vi "Set 2D Next Vector_entwurf.vi"(0 "Coordinate System":u16(ring) items=["Cartesian", "Polar"], 1 "Magnetic Field Units":u16(ring) items=["kG", "Tesla"], 3 "User defined Ramp Rate (T/min)":dbl format="%.3f", 4 "Magnitude Limit (kG)":dbl format="%.3f", 5 "Y-Axis Communications Config":T1={"GPIB address"=22, "GPIB bus"=0, "connection ID"=refnum, "IP"="192.168.2.200", "Active Comm Interface"=0, "Serial Port"="", "Programmer Type"=0} {"Programmer Type" items=["Model 430", "Model 420"]; "Active Comm Interface" items=["TCP/IP (Model 430 Only)", "RS232", "IEEE488"]}, 6 "Input Vector":string[](array[string]), 7 "Z-Axis Communications Config":T1={"GPIB address"=22, "GPIB bus"=0, "connection ID"=refnum, "IP"="192.168.2.200", "Active Comm Interface"=0, "Serial Port"="", "Programmer Type"=0} {"Programmer Type" items=["Model 430", "Model 420"]; "Active Comm Interface" items=["TCP/IP (Model 430 Only)", "RS232", "IEEE488"]}, 10 "User defined Ramp Rate (T/min)":bool, 13 "Max Ramp Rate - Y Axis (A/s)":dbl format="%.3f", 14 "error in":T2, 15 "Max Ramp Rate - Z Axis (A/s)":dbl format="%.3f") -> (11 "Y-Axis Ramp Rate (T/min)":dbl format="%.3f", 12 "Within Limits?":bool, 16 "Ramp Rate along Vector (T/min)":dbl, 17 "Z-Axis Ramp Rate (T/min)":dbl format="%.3f", 18 "All Instruments Responded?":bool, 19 "error out":T2)   [LabVIEW 2016]
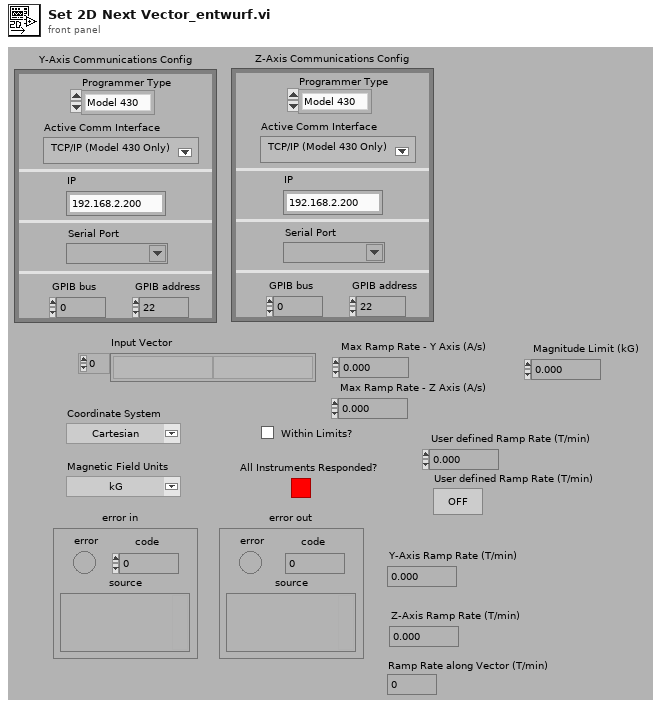
[diagram p1: front panel]
types:
  T1 = cluster{"GPIB address":i16, "GPIB bus":i16, "connection ID":refnum<k5>, "IP":string, "Active Comm Interface":u16, "Serial Port":refnum<visa-resource-name>, "Programmer Type":u16}
  T2 = cluster{"error":bool, "code":i32, "source":string}
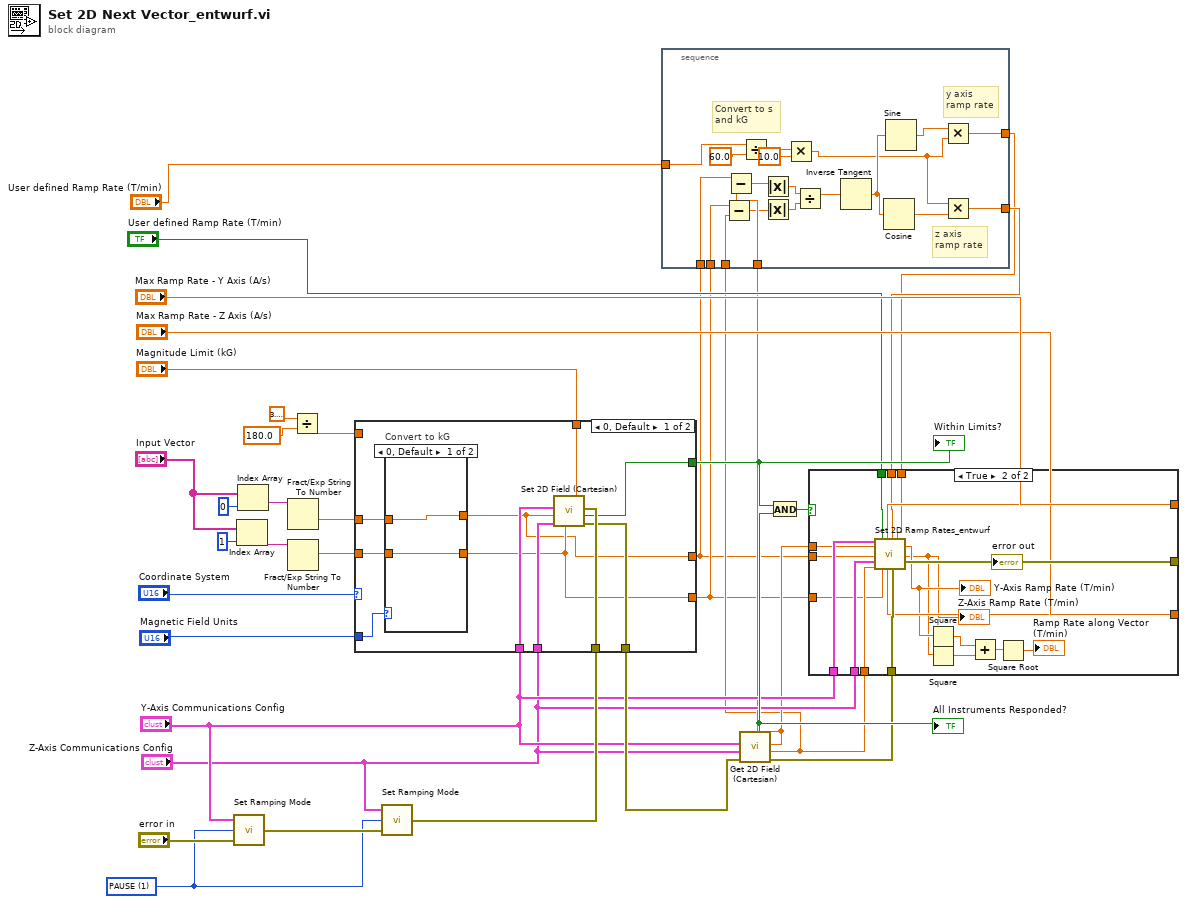
[diagram p0: block diagram]
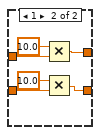
[diagram p3: hidden frame]
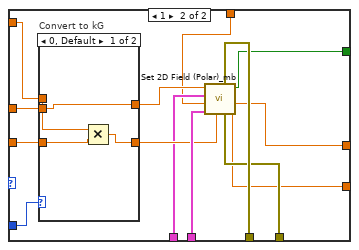
[diagram p4: hidden frame]
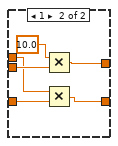
[diagram p5: hidden frame]
diagram:
  w20 = u16 1 items=["RAMP", "PAUSE", "MANUAL UP", "MANUAL DOWN", "ZERO"] ("Ramping Mode")
  n1 = call "Set Ramping Mode.vi"("error in"="error in", "Ramping Mode"=w20, "Communications Config"="Y-Axis Communications Config") -> ("error out"=w21:T2)
  n2 = Index Array(array="Input Vector", index=1 ("Index")) -> (element=w31:string)
  n3 = Index Array(array="Input Vector", index=0 ("Index")) -> (element=w32:string)
  n4 = Fract/Exp String To Number(string=w32) -> (number=w11:dbl)  [unwired: 3 in, 1 out]
  n5 = Fract/Exp String To Number(string=w31) -> (number=w10:dbl)  [unwired: 3 in, 1 out]
  n6 = Divide(x=3.141592653589793, y=180.0) -> (x/y=w8:dbl)
  n7 = call "Set Ramping Mode.vi"("error in"=w21, "Ramping Mode"=w20, "Communications Config"="Z-Axis Communications Config") -> ("error out"=w19:T2)
  n8 = case shown="0, Default" "Coordinate System" {
    tunnel: "Magnetic Field Units" -> [w46 w68]
    tunnel: w11 -> [w45 w67]
    tunnel: w10 -> [w44 w66]
    tunnel: "Y-Axis Communications Config" -> [w43 w57]
    tunnel: "Z-Axis Communications Config" -> [w42 w63]
    tunnel: w19 -> [w41 w64]
    tunnel: [w40 w60] -> w29
    tunnel: [w39 w61] -> w18
    tunnel: [w38 w58] -> w2
    tunnel: [w37 w59] -> w1
    tunnel: w8 -> [_ w65]
    tunnel: "Magnitude Limit (kG)" -> [w36 w55]
    frame 0, Default {
      n9 = case "Convert to kG" shown="0, Default" w46 {
        tunnel: w45 -> [w48 w52]
        tunnel: w44 -> [w47 w51]
        tunnel: [w48 w50] -> w37
        tunnel: [w47 w49] -> w38
        frame 0, Default {
        }
        frame 1 {
          n10 = Multiply(x=10.0, y=w52) -> (x*y=w50:dbl)
          n11 = Multiply(x=10.0, y=w51) -> (x*y=w49:dbl)
        }
      }
      n12 = call "Set 2D Field (Cartesian).vi"("error in"=w41, "Magnitude Limit (T)"=w36, "Z-Axis Field (T)"=w38, "Z-Axis Communications Config"=w42, "Y-Axis Field (T)"=w37, "Y-Axis Communications Config"=w43) -> ("error out"=w39:T2, "Within Limits?"=w40:bool)  [unwired: 2 in]
    }
    frame 1 {
      n13 = case "Convert to kG" shown="0, Default" w68 {
        tunnel: w67 -> [w71 w78]
        tunnel: w66 -> [w70 w77]
        tunnel: [w71 w76] -> w56
        tunnel: [w69 w75] -> w62
        tunnel: w65 -> [w72 w74]
        frame 0, Default {
          n14 = Multiply(x=w72, y=w70) -> (x*y=w69:dbl)
        }
        frame 1 {
          n15 = Multiply(x=10.0, y=w78) -> (x*y=w76:dbl)
          n16 = Multiply(x=w74, y=w77) -> (x*y=w75:dbl)
        }
      }
      n17 = call "Set 2D Field (Polar)_mb.vi"("error in"=w64, "f (radians)"=w62, "Z-Axis Communications Config"=w63, "Magnitude Limit (kG)"=w55, "Y-Axis Communications Config"=w57, "Field Magnitude r (kG)"=w56) -> ("Z-Axis Field (kG) out"=w58:dbl, "Y-Axis Field (kG)"=w59:dbl, "Within Limits?"=w60:bool, "error out"=w61:T2)  [unwired: 2 in]
    }
  }
  "Within Limits?" <- w29
  n18 = call "Get 2D Field (Cartesian).vi"("Z-Axis Communications Config"="Y-Axis Communications Config", 2:"Z-Axis Communications Config", "error in"=w18) -> ("All Instruments Responded?"=w27:bool, "Y-Axis Field (kG)"=w4:dbl, "Z-Axis Field (kG)"=w3:dbl, "error out"=w26:T2)  [unwired: 2 in]
  "All Instruments Responded?" <- w27
  n19 = stacked-sequence {
    tunnel: "User defined Ramp Rate (T/min)" -> [w93]
    tunnel: [w88] -> w6
    tunnel: [w87] -> w7
    tunnel: w4 -> [w86]
    tunnel: w3 -> [w85]
    tunnel: w2 -> [w80]
    tunnel: w1 -> [w79]
    frame #0 {
      # "y axis \nramp rate"
      # "z axis \nramp rate"
      # "Convert to s\nand kG"
      n20 = Subtract(x=w80, y=w85) -> (x-y=w83:dbl)
      n21 = Subtract(x=w79, y=w86) -> (x-y=w84:dbl)
      n22 = Divide(x=w93, y=60.0) -> (x/y=w91:dbl)
      n23 = Absolute Value(x=w84) -> (abs(x)=w81:dbl)
      n24 = Absolute Value(x=w83) -> (abs(x)=w82:dbl)
      n25 = Multiply(x=w91, y=10.0) -> (x*y=w89:dbl)
      n26 = Divide(x=w81, y=w82) -> (x/y=w97:dbl)
      n27 = Inverse Tangent(1:w97) -> (0:w96:dbl)
      n28 = Cosine(x=w96) -> (cos(x)=w94:dbl)
      n29 = Sine(x=w96) -> (sin(x)=w95:dbl)
      n30 = Multiply(x=w95, y=w89) -> (x*y=w88:dbl)
      n31 = Multiply(x=w89, y=w94) -> (x*y=w87:dbl)
    }
  }
  n32 = And(x=w29, y=w27) -> (x .and. y?=w28:bool)
  n33 = case shown="True" w28 {
    tunnel: "Y-Axis Communications Config" -> [_ w117]
    tunnel: "Z-Axis Communications Config" -> [_ w116]
    tunnel: w4 -> [_ w115]
    tunnel: w3 -> [_ w114]
    tunnel: w2 -> [_ w113]
    tunnel: w1 -> [_ w112]
    tunnel: w26 -> [w98 w111]
    tunnel: [w98 w110] -> w25
    tunnel: "Max Ramp Rate - Y Axis (A/s)" -> [_ w109]
    tunnel: "Max Ramp Rate - Z Axis (A/s)" -> [_ w108]
    tunnel: w7 -> [_ w107]
    tunnel: w6 -> [_ w106]
    tunnel: "User defined Ramp Rate (T/min)" -> [_ w105]
    frame False {
    }
    frame True {
      n34 = call "Set 2D Ramp Rates_entwurf.vi"("Y-Axis Communications Config"=w117, "Y-Axis Field (kG)"=w115, "Next Y-Axis Field (kG)"=w112, "Z-Axis Communications Config"=w116, "Z-Axis Field (kG)"=w114, "User defined Ramp Rate (T/min)"=w105, "Next Z-Axis Field (kG)"=w113, "Max Ramp Rate - Y Axis (A/s)"=w109, "Max Ramp Rate - Z Axis (A/s)"=w108, "User defined Ramp Rate - Z Axis (kG/s)"=w107, "error in"=w111, "User defined Ramp Rate Y-Axis (kG/s)"=w106) -> ("Y-Axis Ramp Rate (T/min)"=w104:dbl, "Z-Axis Ramp Rate (T/min)"=w103:dbl, "error out"=w110:T2)  [unwired: 5 in]
      "Y-Axis Ramp Rate (T/min)" <- w104
      "Z-Axis Ramp Rate (T/min)" <- w103
      n35 = Square(x=w104) -> (x^2=w101:dbl)
      n36 = Square(x=w103) -> (x^2=w102:dbl)
      n37 = Add(x=w101, y=w102) -> (x+y=w100:dbl)
      n38 = Square Root(x=w100) -> (sqrt(x)=→"Ramp Rate along Vector (T/min)":dbl)
    }
  }
  "error out" <- w25
